vi "main_VI_one_noRT.vi"() -> ()   [LabVIEW 2019]
uses:
  <vilib>/myRIO/Instrument Drivers/Onboard IO/UART/typedef/VISA Configuration.ctl
  <vilib>/Platform/TimedLoop/XDataNode/timing_clust.ctl
  <vilib>/Platform/TimedLoop/XDataNode/nitl_modes.ctl
  <vilib>/Platform/TimedLoop/XDataNode/wakeup.ctl
  <vilib>/Instr/_visa.llb/VISA Configure Serial Port (Instr).vi
  <vilib>/FPGAPlugInAG/myRIO-1900/niLvFpga_Open_myRIO-1900.vi
  <vilib>/rvi/interface/common/dynamic/niFpgaDynamicAddResources.vi
  <vilib>/Utility/error.llb/Error Cluster From Error Code.vi
  <vilib>/rvi/errors/niLvFpgaAdjustHostInterfaceError.vi
  <vilib>/FPGAPlugInAG/Dynamic/niLvFpga_Close_Dynamic.vi
  <vilib>/rvi/interface/nirviOpenFPGA/nirviOpenFPGA.xnode
  FPGA Bitfiles/imuwired_FPGATarget_FPGAFSR_4dEayfvYof8.lvbitx
  FPGA_FSR.vi
  <vilib>/Platform/TimedLoop/XDataNode/XDataNode.xnode
  <vilib>/rvi/interface/nirviReadWriteControl/nirviReadWriteControl.xnode
  <vilib>/rvi/interface/nirviCloseFPGA/nirviCloseFPGA.xnode
  <vilib>/Platform/TimedLoop/XDataNode/XDNodeRunTimeDep.lvlib
  <vilib>/myRIO/Instrument Drivers/Onboard IO/UART/UART.lvlib
  NiFpgaLv.dll
  <vilib>/rvi/interface/Simulation/niFpgaSimulationCallBeginRW.vi
panel:
  out "ConnectorA/AI3":u16
  out "ConnectorA/AI2":u16
  out "ConnectorA/AI1":u16
  out "ConnectorA/AI0":u16
  out "Time":dbl
  in  "file no.":u32
  in  "stop":bool
  in  "error in":errorcluster
  out "error out":errorcluster
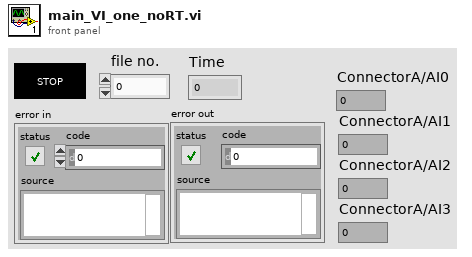
[diagram p1: front panel]
types:
  T1 = enum16{"open", "replace", "create", "open or create", "replace or create", "replace or create with confirmation"}
  T2 = typedef "UART.lvlib/VISA Configuration.ctl" = cluster{"baud rate (9600)":u32, "data bits (8)":u16, "parity (0:none)":enum16{"None", "Odd", "Even", "Mark", "Space"}, "stop bits (10: 1 bit)":u16, "flow control (0:none)":u16, "termination char\n(0xA = '\\n' = LF) ":u8, "Enable Termination\nChar (T)":bool, "timeout (10sec)":u32}
  T3 = typedef "XDNodeRunTimeDep.lvlib/timing_clust.ctl" = cluster{"Expected End [f-1]":u64, "Actual End [f-1]":u64, "Finished Late? [f-1]":bool, "Expected End [i-1]":u64, "Actual End [i-1]":u64, "Finished Late? [i-1]":bool, "Expected Start [i]":u64, "Actual Start [i]":u64, "Expected Start [f]":u64, "Actual Start [f]":u64, "Source Name":string, "Structure Name":string, "Period":i64, "Deadline":i64, "Offset":i64, "Start":i64, "Priority":i32, "Timeout":i32, "Mode":T4, "Wakeup Reason":T5, "Error":errorcluster, "Source Type":string, "Secondary Source Type":string, "Global End Time":u64, "Global Start Time":u64, "Frame Duration":u64, "Iteration Duration":u64, "Assigned CPU":i32, "I/O Scan Engine Mode":u32}
  T4 = typedef "XDNodeRunTimeDep.lvlib/nitl_modes.ctl" = enum32{"No Change", "Process missed periods, maintain original phase", "Discard missed periods, maintain original phase", "Process missed periods, ignore original phase", "Discard missed periods, ignore original phase"}
  T5 = typedef "XDNodeRunTimeDep.lvlib/wakeup.ctl" = enum32{"Normal", "Aborted", "Asynchronous wakeup", "Timing source error", "Timed loop error", "Timeout"}
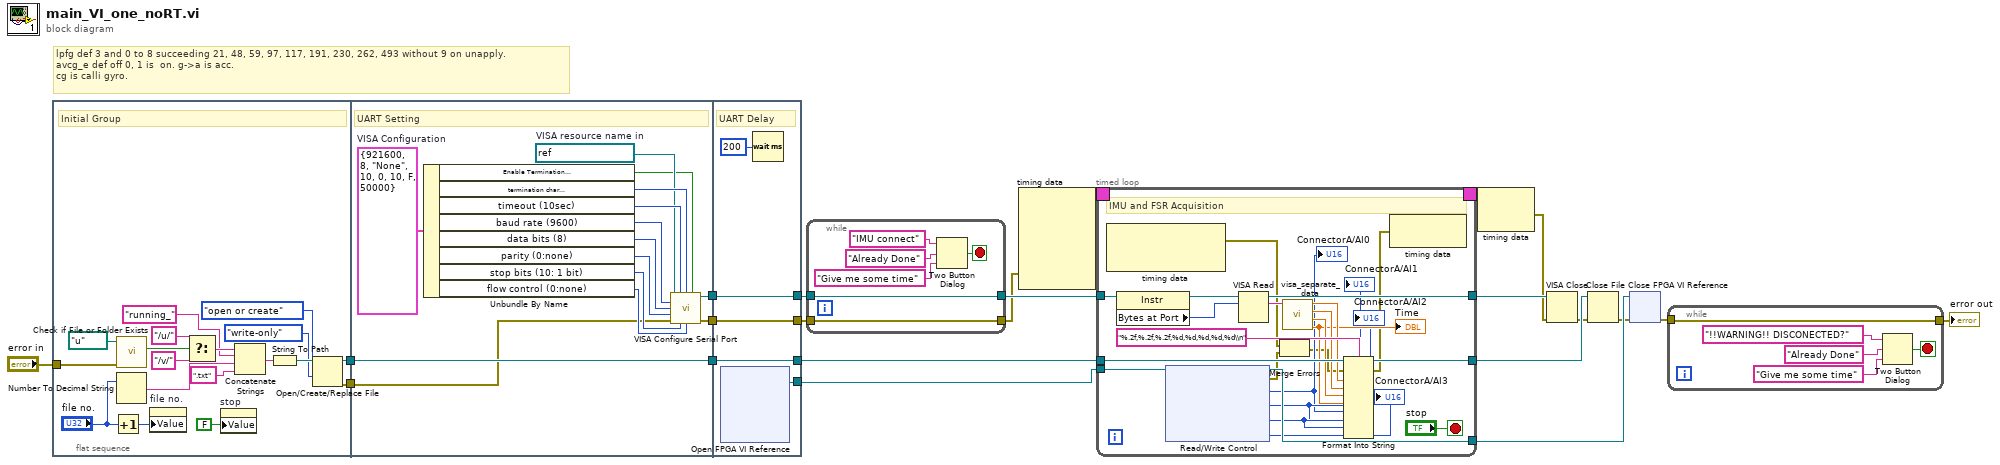
[diagram p0: block diagram]
diagram:
  # "lpfg def 3 and 0 to 8 succeeding 21, 48, 59, 97, 117, 191, 230, 262, 493 without 9 on unapply.\navcg_e def off 0, 1 is  on. g->a is acc.\ncg is calli gyro."
  n1 = flat-sequence {
    tunnel: "error in" -> [w24]
    tunnel: [w25] -> w8
    tunnel: [w23] -> w7
    tunnel: w8 -> [w54]
    tunnel: w7 -> [w44]
    tunnel: [w54] -> w4
    tunnel: [w43] -> w3
    tunnel: [w42] -> w2
    tunnel: [w57] -> w5
    tunnel: [w58] -> w6
    tunnel: [w59] -> w10
    tunnel: w4 -> [w59]
    tunnel: w3 -> [w58]
    tunnel: w2 -> [w57]
    tunnel: [w55] -> w1
    frame #0 {
      # "Initial Group"
      n2 = Increment(x="file no.") -> (x+1=w38:u32)
      n3 = call <vilib>:"Check if File or Folder Exists.vi"("error in (no error)"=w24, "path"=path "u:/") -> ("file or folder exists?"=w33:bool)  [unwired: 7 in, 2 out]
      n4 = Number To Decimal String(number="file no.") -> (decimal integer string=w37:string)  [unwired: 1 in]
      n5 = property on="file no." class="DigNum (strict)"("Value"=w38) -> ()  [unwired: 2 in, 2 out]
      n6 = Select(t="/u/", s=w33, f="/v/") -> (s? t:f=w35:string)
      n7 = property on="stop" class="Bool (strict)"("Value"=FALSE ("stop")) -> ()  [unwired: 2 in, 2 out]
      n8 = Concatenate Strings(w35, "running_" ("string"), w37, ".txt" ("string")) -> (w36:string)
      n9 = String To Path(string=w36) -> (path=w34:path)
      n10 = Open/Create/Replace File(file path (use dialog)=w34, operation (0:open)=T1."open or create", access (0:read/write)=enum16{"read/write", "read-only", "write-only"}."write-only") -> (refnum out=w25:refnum<file>, error out=w23:errorcluster)  [unwired: 3 in, 1 out]
    }
    frame #1 {
      w46 = T2 {"baud rate (9600)"=921600, "data bits (8)"=8, "parity (0:none)"=enum."None", "stop bits (10: 1 bit)"=10, "flow control (0:none)"=0, "termination char\n(0xA = '\\n' = LF) "=10, "Enable Termination\nChar (T)"=FALSE, "timeout (10sec)"=50000}  # VISA Configuration
      w45 = refnum<visa-resource-name> "ASRL1::INSTR"  # VISA resource name in
      # "UART Setting"
      n11 = Unbundle By Name(w46) -> ("Enable Termination\nChar (T)"=w41:bool, "termination char\n(0xA = '\\n' = LF)"=w47:u8, "timeout (10sec)"=w48:u32, "baud rate (9600)"=w52:u32, "data bits (8)"=w51:u16, "parity (0:none)"=w50:enum16{"None", "Odd", "Even", "Mark", "Space"}, "stop bits (10: 1 bit)"=w49:u16, "flow control (0:none)"=w53:u16)
      n12 = call-poly "VISA Configure Serial Port"("VISA resource name"=w45, "timeout (10sec)"=w48, "termination char\n(0xA = '\\n' = LF)"=w47, "Enable Termination\nChar (T)"=w41, "baud rate (9600)"=w52, "data bits (8)"=w51, "parity (0:none)"=w50, "error in (no error)"=w44, "stop bits (10: 1 bit)"=w49, "flow control (0:none)"=w53) -> ("VISA resource name out"=w43:refnum<visa-resource-name>, "error out"=w42:errorcluster)  [unwired: 4 in]
    }
    frame #2 {
      # "UART Delay"
      n13 = xnode ("Open FPGA VI Reference")() -> ("FPGA VI Reference Out"=w55:refnum<k20>)  [unwired: 2 in, 1 out]
      n14 = Wait (ms)(milliseconds to wait=u32 200) -> ()  [unwired: 1 out]
    }
  }
  n15 = while {
    tunnel: [w65] -> w16
    tunnel: w5 -> [w65]
    tunnel: [w64] -> w18
    tunnel: w6 -> [w64]
    stop <- w60 stop-if-true
    n16 = Two Button Dialog(message="IMU connect", 1:"Give me some time" ("F button name (\"Cancel\")"), 2:"Already Done" ("button name (\"OK\")")) -> (T button?=w60:bool)
  }
  n17 = node-c288(w16) -> (w22:T3)  [unwired: 4 in]
  n18 = timed-loop {
    timing: w22 -> [_]
    timing-out: [_] -> w21
    tunnel: w18 -> [w85]
    tunnel: [w88] -> w20
    tunnel: w1 -> [w82]
    tunnel: [w81] -> w15
    tunnel: w10 -> [w79]
    tunnel: [w78] -> w14
    stop <- "stop" stop-if-true
    # "IMU and FSR Acquisition"
    n19 = node-c288() -> (w66:errorcluster)  [unwired: 1 in, 1 out]
    n20 = property class="Instr"(reference=w85) -> (reference out=w84:refnum<visa-resource-name>, "Bytes at Port"=w83:u32)  [unwired: 1 in, 1 out]
    n21 = xnode "Read/Write Control"("FPGA VI Reference In"=w82) -> ("FPGA VI Reference Out"=w81:refnum<k20>, "error out"=w67:errorcluster, "ConnectorA/AI0"=w70:u16, "ConnectorA/AI1"=w71:u16, "ConnectorA/AI2"=w73:u16, "ConnectorA/AI3"=w72:u16)  [unwired: 1 in]
    "ConnectorA/AI0" <- w70
    "ConnectorA/AI1" <- w71
    "ConnectorA/AI2" <- w73
    "ConnectorA/AI3" <- w72
    n22 = VISA Read(VISA resource name=w84, byte count=w83) -> (VISA resource name out=w88:refnum<visa-resource-name>, read buffer=w87:string)  [unwired: 1 in, 2 out]
    n23 = Merge Errors(w66, w67) -> (w68:errorcluster)
    n24 = call "visa_separate_data.vi"("Input string"=w87) -> ("Time"=w74:dbl, "Gyro_z"=w76:dbl, "Gyro_y"=w75:dbl, "Gyro_x"=w77:dbl)  [unwired: 7 in]
    "Time" <- w74
    n25 = Format Into String(format string="%.2f,%.2f,%.2f,%d,%d,%d,%d,%d\\n", initial string=w79, error in=w68, w77, w75, w76, w74, w70, w71, w73, w72) -> (resulting string=w78:refnum<file>, error out=w69:errorcluster)
    n26 = node-c288(w69) -> ()  [unwired: 1 out]
  }
  n27 = node-c288(w21) -> (w12:errorcluster)
  n28 = VISA Close(VISA resource name=w20, error in (no error)=w12) -> (error out=w11:errorcluster)
  n29 = Close File(refnum=w14, error in=w11) -> (error out=w9:errorcluster)  [unwired: 1 out]
  n30 = xnode "Close FPGA VI Reference"("FPGA VI Reference In"=w15, "error in"=w9) -> ("error out"=w13:errorcluster)
  n31 = while {
    tunnel: [w98] -> w19
    tunnel: w13 -> [w98]
    stop <- w94 stop-if-true
    n32 = Two Button Dialog(message="!!WARNING!! DISCONECTED?", 1:"Give me some time" ("F button name (\"Cancel\")"), 2:"Already Done" ("button name (\"OK\")")) -> (T button?=w94:bool)
  }
  "error out" <- w19
